vi "7 segement led.vi"() -> ()   [LabVIEW 2018]
panel:
  in  "Numeric":dbl
  out "?":bool
  out "?":bool
  out "?":bool
  out "?":bool
  out "?":bool
  out "?":bool
  out "?":bool
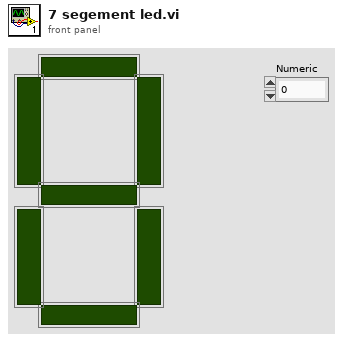
[diagram p1: front panel]
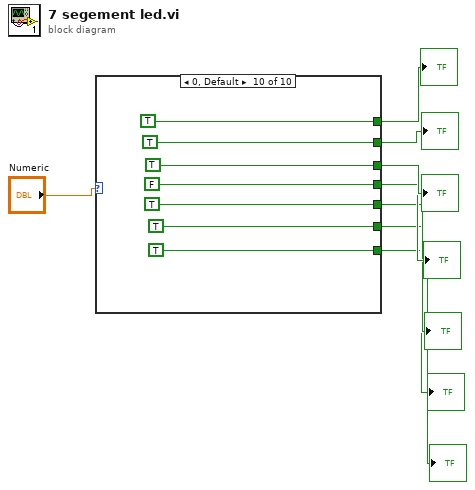
[diagram p0: block diagram]
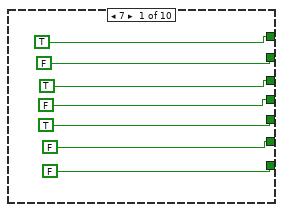
[diagram p2: hidden frame]
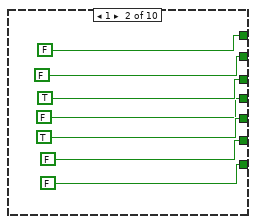
[diagram p3: hidden frame]
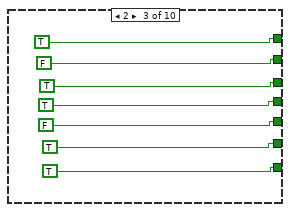
[diagram p4: hidden frame]
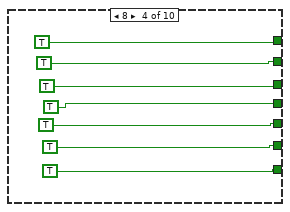
[diagram p5: hidden frame]
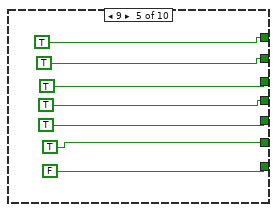
[diagram p6: hidden frame]
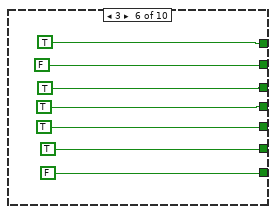
[diagram p7: hidden frame]
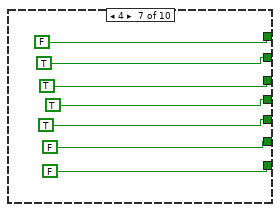
[diagram p8: hidden frame]
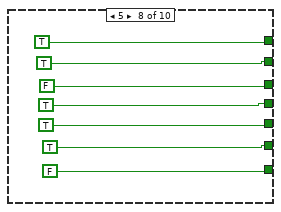
[diagram p9: hidden frame]
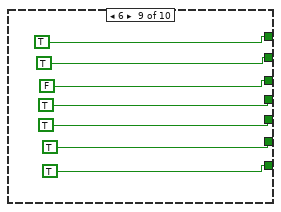
[diagram p10: hidden frame]
diagram:
  n1 = case shown="0, Default" "Numeric" {
    tunnel: [TRUE FALSE TRUE TRUE TRUE TRUE FALSE TRUE TRUE TRUE] -> w7
    tunnel: [FALSE FALSE FALSE TRUE TRUE FALSE TRUE TRUE TRUE TRUE] -> w6
    tunnel: [TRUE TRUE TRUE TRUE TRUE TRUE TRUE FALSE FALSE TRUE] -> w5
    tunnel: [FALSE FALSE TRUE TRUE TRUE TRUE TRUE TRUE TRUE FALSE] -> w4
    tunnel: [TRUE TRUE FALSE TRUE TRUE TRUE TRUE TRUE TRUE TRUE] -> w3
    tunnel: [FALSE FALSE TRUE TRUE TRUE TRUE FALSE TRUE TRUE TRUE] -> w2
    tunnel: [FALSE FALSE TRUE TRUE FALSE FALSE FALSE FALSE TRUE TRUE] -> w1
    frame 7 {
    }
    frame 1 {
    }
    frame 2 {
    }
    frame 8 {
    }
    frame 9 {
    }
    frame 3 {
    }
    frame 4 {
    }
    frame 5 {
    }
    frame 6 {
    }
    frame 0, Default {
    }
  }
  "?" <- w7
  "?" <- w6
  "?" <- w5
  "?" <- w4
  "?" <- w3
  "?" <- w2
  "?" <- w1
